vi "Validate_Local_Destination.vi"(8 "error in (no error)":errorcluster, 11 "AB_Build in":refnum<class "AB_Build.lvclass">) -> (0 "error out":errorcluster, 3 "AB_Build out":refnum<class "AB_Build.lvclass">)   [LabVIEW 2020, in "AB_Build.lvclass"]
uses:
  <vilib>/AppBuilder/AB_Classes/Build/AB_Build.lvclass
  <vilib>/AppBuilder/AB_Classes/Build/AB_Build.lvclass/AB_Build.ctl
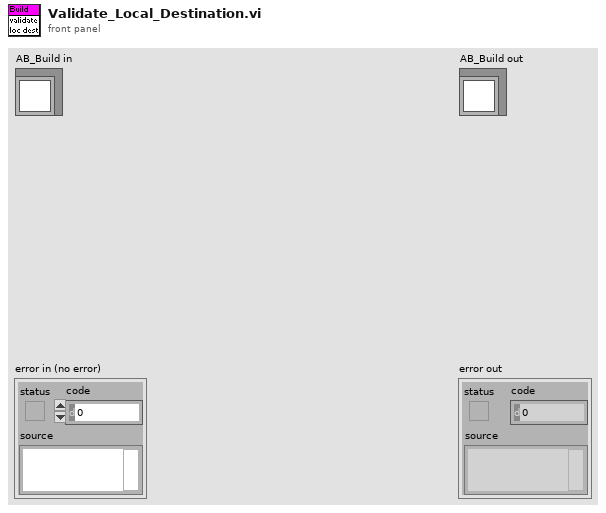
[diagram p1: front panel]
types:
  T1 = typedef "ItemRef.ctl" = u64
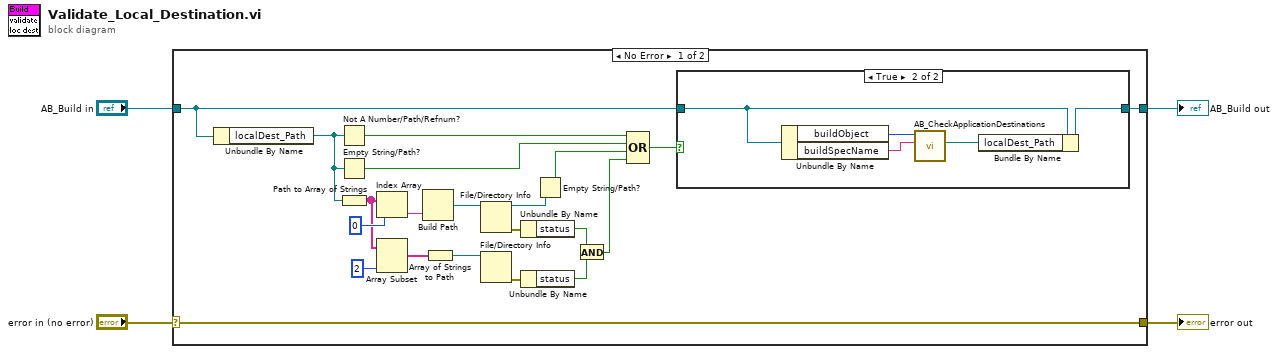
[diagram p0: block diagram]
diagram:
  n1 = case shown="No Error" "error in (no error)" {
    selector: "error in (no error)" -> [w25 w33]
    tunnel: [w25 w33] -> w3
    tunnel: [w6 w32] -> w2
    tunnel: "AB_Build in" -> [w5 w32]
    frame No Error {
      n2 = Unbundle By Name(w5) -> ("localDest_Path"=w8:path)
      n3 = Not A Number/Path/Refnum?(number/path/refnum=w8) -> (NaN/Path/Refnum?=w20:bool)
      n4 = Empty String/Path?(string/path=w8) -> (empty?=w19:bool)
      n5 = Path to Array of Strings(0:w8) -> (2:w17:string[])  [unwired: 1 out]
      n6 = Index Array(array=w17, index=0) -> (element=w22:string)
      n7 = Array Subset(array=w17, length=2) -> (w15:string[])  [unwired: 1 in]
      n8 = Build Path(name or relative path=w22) -> (appended path=w21:path)  [unwired: 1 out]
      n9 = Array of Strings to Path(0:w15) -> (2:w13:path)  [unwired: 1 out]
      n10 = File/Directory Info(path=w21) -> (path out=w10:path, error out=w24:errorcluster)  [unwired: 1 in, 5 out]
      n11 = File/Directory Info(path=w13) -> (error out=w14:errorcluster)  [unwired: 1 in, 6 out]
      n12 = Unbundle By Name(w24) -> ("status"=w12:bool)
      n13 = Unbundle By Name(w14) -> ("status"=w11:bool)
      n14 = Empty String/Path?(string/path=w10) -> (empty?=w18:bool)
      n15 = And(x=w12, y=w11) -> (x .and. y?=w9:bool)
      n16 = Compound Arithmetic op=OR(w20, w19, w18, w9) -> (w7:bool)
      n17 = case shown="True" w7 {
        tunnel: w5 -> [w26 w27]
        tunnel: [w26 w31] -> w6
        frame False {
        }
        frame True {
          n18 = Unbundle By Name(w27) -> ("buildObject"=w30:T1, "buildSpecName"=w29:string)
          n19 = call <vilib>:"AB_CheckApplicationDestinations.vi"("buildSpecName"=w29, "buildObject"=w30) -> ("Checked base path"=w28:path)  [unwired: 3 in, 6 out]
          n20 = Bundle By Name(cluster=w27, "localDest_Path"=w28) -> (w31:refnum<class "AB_Build.lvclass">)
        }
      }
    }
    frame Error {
    }
  }
  "error out" <- w3
  "AB_Build out" <- w2
